vi "配置文件写入.vi"(8 "error in (no error)":errorcluster caption="错误输入（无错误）") -> (0 "错误输出":errorcluster)   [LabVIEW 2016]
uses:
  <vilib>/Utility/config.llb/NI_LVConfig.lvlib
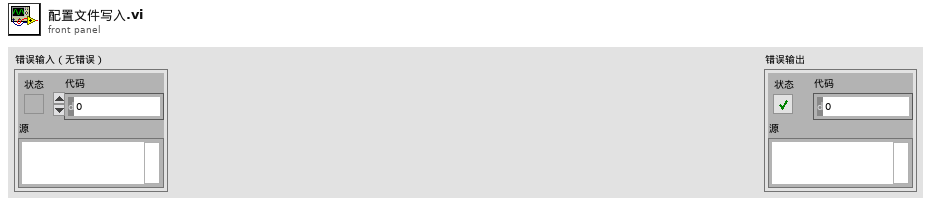
[diagram p1: front panel]
types:
  T1 = typedef "NI_LVConfig.lvlib/Config Data RefNum.ctl" = refnum<k1>
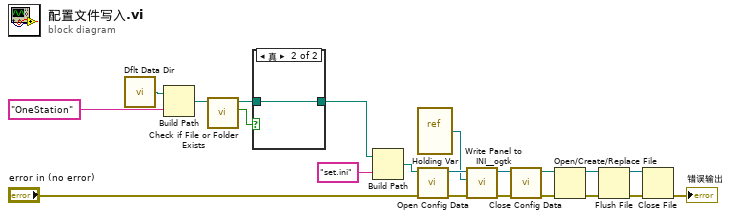
[diagram p0: block diagram]
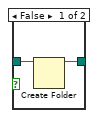
[diagram p2: hidden frame]
diagram:
  n1 = call <vilib>:"Dflt Data Dir.vi"() -> ("App:Default Data Directory"=w20:path)
  n2 = Build Path(base path=w20, name or relative path="OneStation" ("名称或相对路径")) -> (appended path=w18:path)
  n3 = call <vilib>:"Check if File or Folder Exists.vi"("path"=w18) -> ("file or folder exists?"=w17:bool, "dup path"=w16:path)  [unwired: 8 in, 1 out]
  n4 = case shown="真" w17 {
    tunnel: w16 -> [w23 w24]
    tunnel: [w22 w24] -> w15
    frame False {
      n5 = Create Folder(path (use dialog)=w23) -> (created path=w22:path)  [unwired: 2 in, 2 out]
    }
    frame True {
    }
  }
  n6 = Build Path(base path=w15, name or relative path="set.ini" ("名称或相对路径")) -> (appended path=w14:path)
  n7 = vi-ref "Holding Var.vi"() -> (w9:refnum<vi>)
  n8 = call <vilib>:"Open Config Data.vi"("error in (no error)"="error in (no error)", "configuration file path"=w14) -> ("error out"=w13:errorcluster, "refnum"=w12:T1)  [unwired: 7 in, 1 out]
  n9 = call <userlib>:"Write Panel to INI__ogtk.vi"("error in (no error)"=w13, "VI ref"=w9, "refnum"=w12) -> ("error out"=w11:errorcluster, "refnum out"=w10:T1)  [unwired: 7 in]
  n10 = call <vilib>:"Close Config Data.vi"("error in (no error)"=w11, "refnum"=w10) -> ("error out"=w4:errorcluster, "file path"=w3:path)  [unwired: 8 in]
  n11 = Open/Create/Replace File(file path (use dialog)=w3, error in=w4) -> (refnum out=w7:refnum<file>, error out=w8:errorcluster)  [unwired: 4 in, 1 out]
  n12 = Flush File(refnum=w7, error in=w8) -> (refnum out=w6:refnum<file>, error out=w5:errorcluster)
  n13 = Close File(refnum=w6, error in=w5) -> (error out=→"错误输出":errorcluster)  [unwired: 1 out]
